vi "利用单位计算矩形周长与面积.vi"() -> ()   [LabVIEW 2012]
panel:
  out "周长":dbl[unit]
  out "面积":dbl[unit]
  in  "宽度":dbl[unit](slide) scale=0.0..10.0
  in  "长度":dbl[unit](slide) scale=0.0..20.0
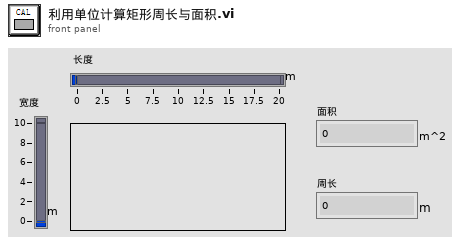
[diagram p1: front panel]
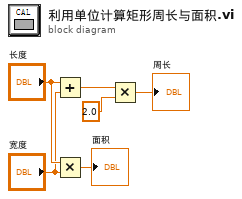
[diagram p0: block diagram]
diagram:
  n1 = Add(x="长度", y="宽度") -> (x+y=w3:dbl[unit])
  n2 = Multiply(x="长度", y="宽度") -> (x*y=→"面积":dbl[unit])
  n3 = Multiply(x=w3, y=2.0) -> (x*y=→"周长":dbl[unit])
